vi "GetParameterByName.vi"(8 "error in (no error)":errorcluster, 10 "Name":string, 11 "Parameter in":refnum<class "Parameter.lvclass">[](array[class])) -> (0 "error out":errorcluster, 2 "Found":bool, 3 "Parameter out":refnum<class "Parameter.lvclass">)   [LabVIEW 2023, in "Easy.SequenceManagerLabVIEW.lvlib" / "Parameter.lvclass"]
uses:
  Parameter.lvclass
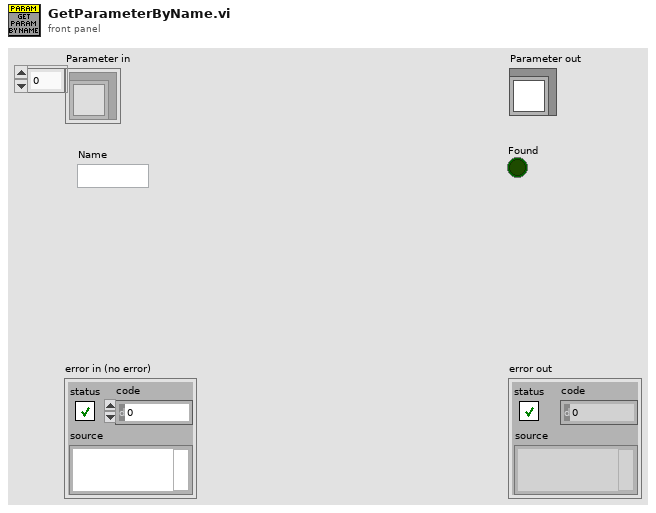
[diagram p1: front panel]
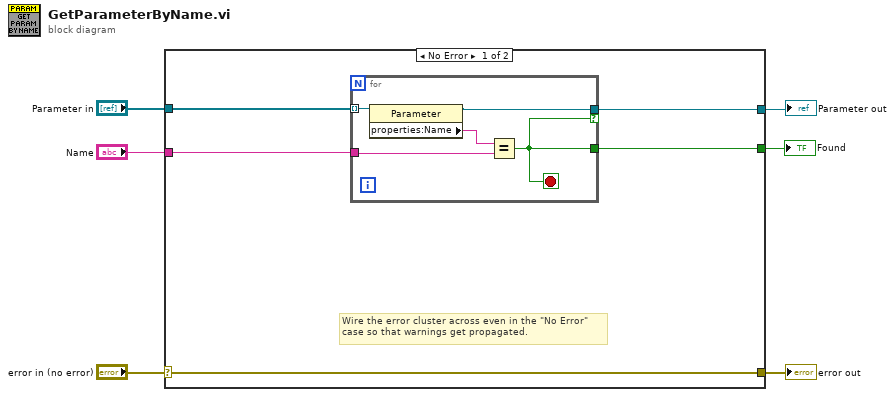
[diagram p0: block diagram]
diagram:
  n1 = case shown="No Error" "error in (no error)" {
    selector: "error in (no error)" -> [w11 w17]
    tunnel: [w11 w17] -> w5
    tunnel: "Parameter in" -> [w10 _]
    tunnel: "Name" -> [w9 _]
    tunnel: [w8 _] -> w2
    tunnel: [w7 _] -> w1
    frame No Error {
      # "Wire the error cluster across even in the \"No Error\"\ncase so that warnings get propagated."
      n2 = for {
        tunnel: w9 -> [w15]
        tunnel: w10 -> [w16] mode=indexing
        tunnel: [w13] -> w8 if=w12
        tunnel: [w12] -> w7
        stop <- w12 stop-if-true
        n3 = property class="Parameter"(reference=w16) -> (reference out=w13:refnum<class "Parameter.lvclass">, "properties:Name"=w14:string)  [unwired: 1 in, 1 out]
        n4 = Equal?(x=w14, y=w15) -> (x = y?=w12:bool)
      }
    }
    frame Error {
    }
  }
  "error out" <- w5
  "Parameter out" <- w2
  "Found" <- w1
